vi "Init.vi"(8 "error in (no error)":errorcluster, 10 "Blueprint String":string, 11 "Robots in":refnum<class "Blueprint.lvclass">) -> (0 "error out":errorcluster, 3 "Robots out":refnum<class "Blueprint.lvclass">)   [LabVIEW 2021, in "d19.lvlib" / "Blueprint.lvclass"]
uses:
  Blueprint/Blueprint.lvclass
  Blueprint/Blueprint.lvclass/Blueprint.ctl
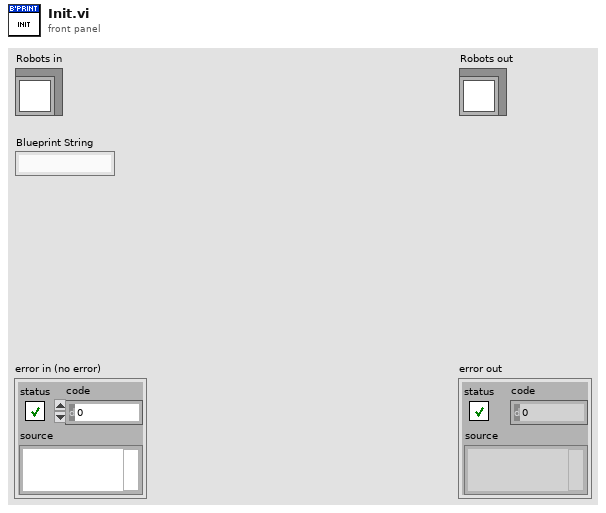
[diagram p1: front panel]
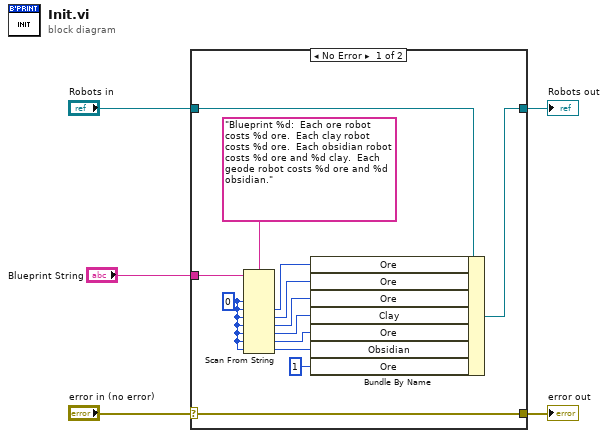
[diagram p0: block diagram]
diagram:
  n1 = case shown="No Error" "error in (no error)" {
    selector: "error in (no error)" -> [w18 w20]
    tunnel: [w18 w20] -> w4
    tunnel: [w15 w19] -> w2
    tunnel: "Robots in" -> [w14 w19]
    tunnel: "Blueprint String" -> [w17 _]
    frame No Error {
      w7 = i64 0 ("default value 1")
      n2 = Scan From String(format string="Blueprint %d:  Each ore robot costs %d ore.  Each clay robot costs %d ore.  Each obsidian robot costs %d ore and %d clay.  Each geode robot costs %d ore and %d obsidian.", input string=w17, default 1=w7, default 2=w7, default 3=w7, default 4=w7, default 5=w7, default 6=w7, default 7=w7) -> (output 2=w13:i64, output 3=w12:i64, output 4=w11:i64, output 5=w10:i64, output 6=w9:i64, output 7=w8:i64)  [unwired: 3 in, 3 out]
      n3 = Bundle By Name(cluster=w14, "Ore"=w13, "Ore"=w12, "Ore"=w11, "Clay"=w10, "Ore"=w9, "Obsidian"=w8, "Ore"=u64 1 ("Robots.Ore")) -> (w15:refnum<class "Blueprint.lvclass">)
    }
    frame Error {
    }
  }
  "error out" <- w4
  "Robots out" <- w2
